vi "GenerateFoodPosition.vi"(10 "Food Amount":i32) -> (2 "Food Array":i32[][](array[numeric]))   [LabVIEW 2021]
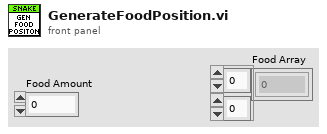
[diagram p1: front panel]
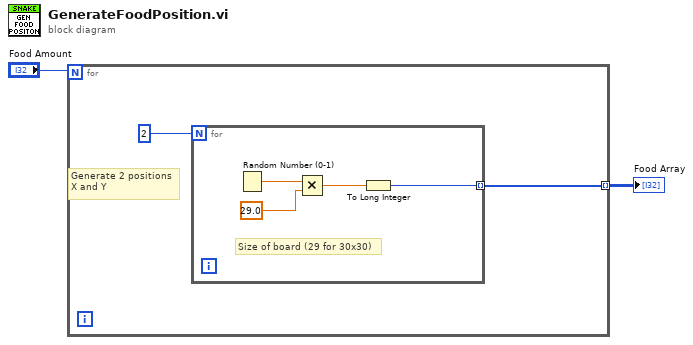
[diagram p0: block diagram]
diagram:
  n1 = for {
    N: "Food Amount" -> [_]
    tunnel: [w3] -> w1 mode=indexing
    # "Generate 2 positions\nX and Y"
    n2 = for {
      N: 2 -> [_]
      tunnel: [w5] -> w3 mode=indexing
      # "Size of board (29 for 30x30)"
      n3 = Random Number (0-1)() -> (number: 0 to 1=w8:dbl)
      n4 = Multiply(x=w8, y=29.0) -> (x*y=w6:dbl)
      n5 = To Long Integer(number=w6) -> (32bit integer=w5:i32)
    }
  }
  "Food Array" <- w1
